vi "De-Initialize.vi"(8 "error in (no error)":errorcluster, 11 "ZI Lockin in":refnum<class "ZI Lockin.lvclass">) -> (0 "error out":errorcluster, 3 "ZI Lockin out":refnum<class "ZI Lockin.lvclass">)   [LabVIEW 2016, in "ZI Lockin.lvclass"]
uses:
  ZI Lockin.lvclass
  ZI Lockin.lvclass/ZI Lockin.ctl
  Read ZI Handle.vi
  Write ZI Handle.vi
  Program Files/National Instruments/LabVIEW 2016/instr.lib/Zurich Instruments LabOne/Zurich Instruments LabOne.lvlib
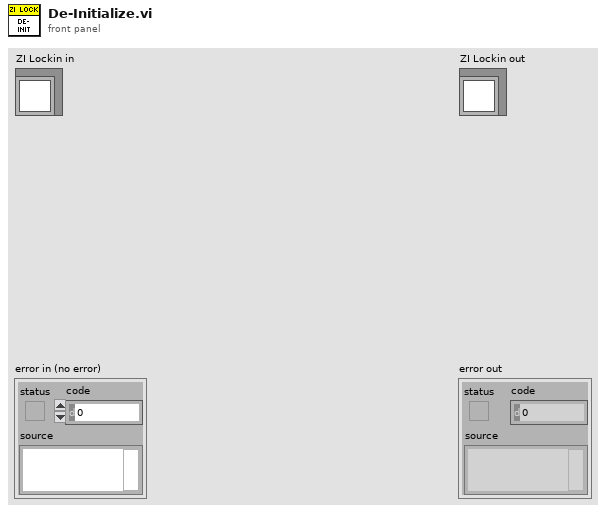
[diagram p1: front panel]
types:
  T1 = typedef "Zurich Instruments LabOne.lvlib/ziTypeHandle.ctl" = cluster{"handleValid":bool, "Conn":u64, "Path Prefix":string, "Handle":u64, "Connected":bool, "Clockbase(s)":dbl}
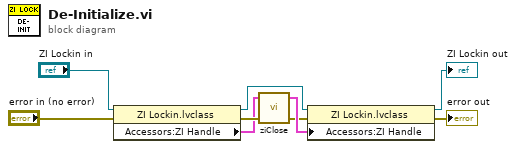
[diagram p0: block diagram]
diagram:
  n1 = property class="ZI Lockin.lvclass"(reference="ZI Lockin in", error in="error in (no error)") -> (reference out=w9:refnum<class "ZI Lockin.lvclass">, error out=w7:errorcluster, "Accessors:ZI Handle"=w1:T1)
  n2 = call "ziClose.vi"("Error In"=w7, "Handle In"=w1) -> ("Error Out"=w6:errorcluster, "Handle Out"=w8:T1)  [unwired: 2 in]
  n3 = property class="ZI Lockin.lvclass"(reference=w9, error in=w6, "Accessors:ZI Handle"=w8) -> (reference out=→"ZI Lockin out":refnum<class "ZI Lockin.lvclass">, error out=→"error out":errorcluster)
